vi "Coloring Doppler Demo.vi"() -> ()   [LabVIEW 2018]
uses:
  user.lib/SpectralRadar.llb/OCT Device.lvclass
  user.lib/SpectralRadar.llb/Probe.lvclass
  user.lib/SpectralRadar.llb/Processing.lvclass
  user.lib/SpectralRadar.llb/Raw Data.lvclass
  user.lib/SpectralRadar.llb/Scan Pattern.lvclass
  user.lib/SpectralRadar.llb/Coloring.lvclass
  user.lib/SpectralRadar.llb/Colored Data.lvclass
  user.lib/SpectralRadar.llb/Coloring Byteorder.ctl
  user.lib/SpectralRadar.llb/Device Camera Preset Selection.ctl
  user.lib/SpectralRadar.llb/LabVIEW Helper.lvlib
  user.lib/SpectralRadar.llb/Processing Parameter Int Selection.ctl
  user.lib/SpectralRadar.llb/Colored Data Export Format Selection.ctl
  user.lib/SpectralRadar.llb/set Complex Scan Output.vi
  user.lib/SpectralRadar.llb/Colorscheme Selection.ctl
  user.lib/SpectralRadar.llb/Complex Data.lvclass
  user.lib/SpectralRadar.llb/Doppler Processing.lvclass
  user.lib/SpectralRadar.llb/set Doppler Phase Output.vi
  user.lib/SpectralRadar.llb/set Doppler Amplitude Output.vi
  user.lib/SpectralRadar.llb/Doppler Property Int.ctl
  user.lib/SpectralRadar.llb/Data.lvclass
panel:
  in  "Averaging Z":i32=1
  in  "Averaging X":i32=2 min=2 max=20 step=1
  in  "Min Signal [dB]":sgl(slide)=1.4419259 min=-20 max=120 scale=-20.0..120.0
  in  "Doppler Boundaries":cluster{sgl, sgl}(slide)={1.4419259, -0.7006223} scale=-3.1415..3.1415
  in  "Save Button":bool
  in  "File Name":path
  in  "Display On/Off":bool=TRUE
  in  "Range":dbl=1.0
  in  "Color Table Selection":T1
  out "Averaged Frame Rate":dbl=6.134969234466553 format="%#_3g"
  out "Current Frame Rate":dbl=6.134969234466553 format="%#_3g"
  in  "Boundries":cluster{sgl, sgl}(slide)={76.65738, 42.00557} scale=-20.0..120.0
  out "Image":T2(plugin-control)
  in  "stop":bool
  in  "AScans":i32=1024
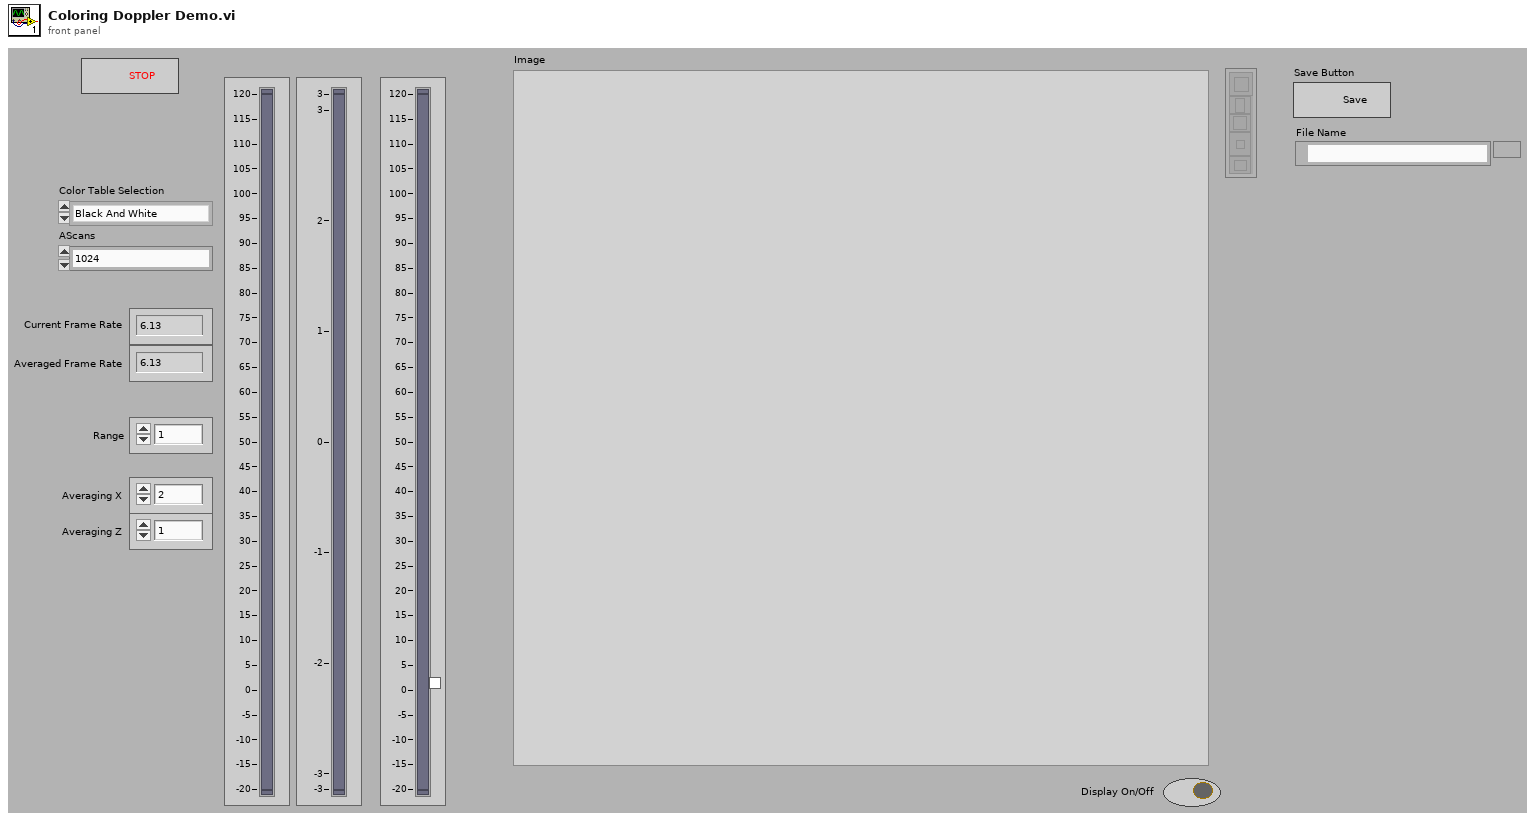
[diagram p1: front panel]
types:
  T1 = typedef "Coloring.lvclass/Colorscheme Selection.ctl" = enum16{"Black And White", "Inverted Black And White", "Color", "Black and Orange", "Black and Red", "Doppler Phase Coloring"}
  T2 = typedef "IMAQ Image.ctl" = refnum<image>
  T3 = typedef "Coloring.lvclass/Coloring Byteorder.ctl" = enum16{"RGBA32", "BGRA32", "ARGB32", ""}
  T4 = typedef "Processing.lvclass/Processing Parameter Int Selection.ctl" = enum32{"Spectrum Averaging", "A-Scan Averaging", "B-Scan Averaging", "Zero Padding", "Number of Threads", "Fourier Averaging"}
  T5 = typedef "OCT Device.lvclass/Device Camera Preset Selection.ctl" = enum16{"Default", "Preset 1", "Preset 2", "Preset 3"}
  T6 = typedef "Image Type" = u32
  T7 = enum16{"Asynchronous Continuous", "Asynchronous Finite", "Synchronous"}
  T8 = typedef "Doppler Processing.lvclass/Doppler Property Int.ctl" = enum16{"Doppler Averaging 1", "Doppler Averaging 2"}
  T9 = typedef "Colored Data.lvclass/Colored Data Export Format Selection.ctl" = enum16{"SRM (Spectral Radar Metafile)", "RAW", "BMP", "PNG", "JPG", "PDF", "TIFF"}
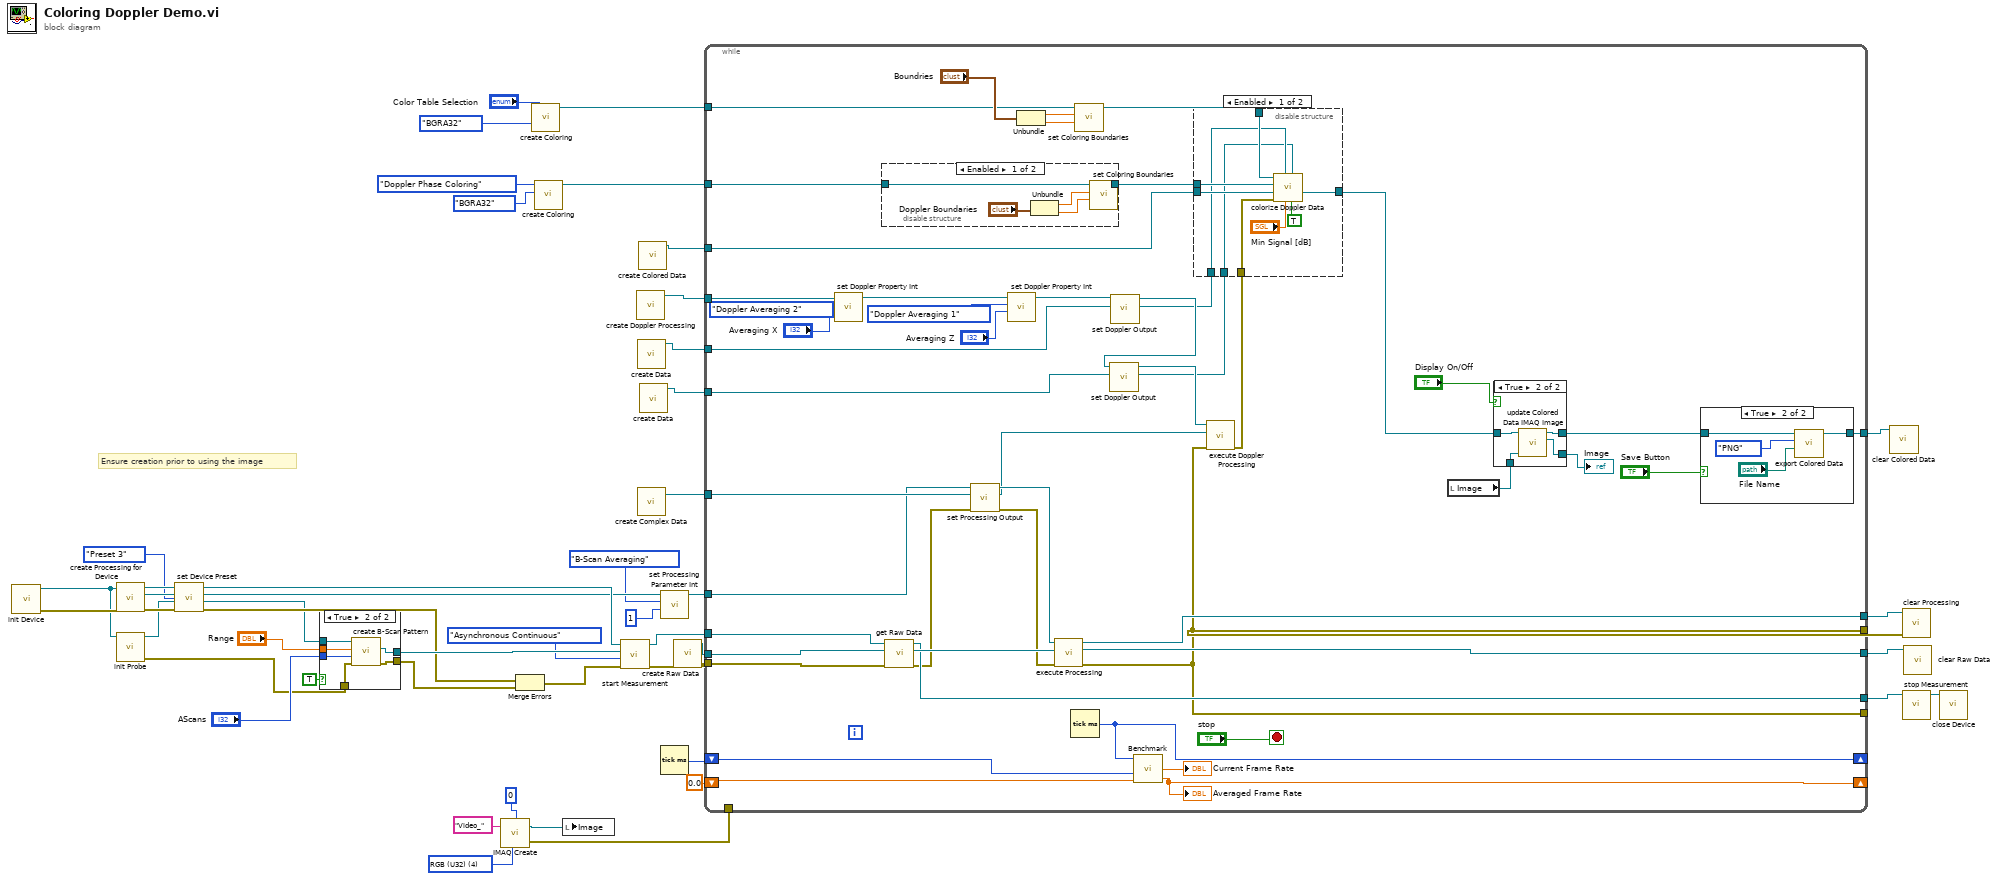
[diagram p0: block diagram]
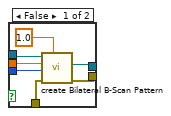
[diagram p2: hidden frame]
diagram:
  w30 = T6 4 items=["Grayscale (U8)", "Grayscale (I16)", "Grayscale (SGL)", "Complex (CSG)", "RGB (U32)", "HSL (U32)", "RGB (U64)", "Grayscale (U16)"] ("Image Type")
  # "Ensure creation prior to using the image"
  n1 = call "init Device.vi"() -> ("error out"=w49:errorcluster, "OCTDevice"=w19:refnum<class "OCT Device.lvclass">)  [unwired: 6 in]
  n2 = call "create Processing for Device.vi"("error in (no error)"=w49, "OCTDevice"=w19) -> ("error out"=w43:errorcluster, "Processing"=w23:refnum<class "Processing.lvclass">, "OCTDevice"=w24:refnum<class "OCT Device.lvclass">)  [unwired: 3 in]
  n3 = call "init Probe.vi"("OCT Device [In]"=w19) -> ("error out"=w32:errorcluster, "OCT Device [Out]"=w20:refnum<class "OCT Device.lvclass">)  [unwired: 4 in, 1 out]
  n4 = call "set Device Preset.vi"("Numeric"=Device_Camera_Preset_Selection."Preset 3" ("Device Camera Preset Selection"), "Probe"=w20, "Processing"=w23, "OCTDevice"=w24) -> ("Probe 2"=w18:refnum<class "Probe.lvclass">, "Processing"=w14:refnum<class "Processing.lvclass">, "OCTDevice out"=w22:refnum<class "OCT Device.lvclass">)  [unwired: 2 in, 1 out]
  n5 = case shown="True" TRUE {
    tunnel: "AScans" -> [w55 w62]
    tunnel: [w54 w61] -> w47
    tunnel: [w53 w60] -> w45
    tunnel: w32 -> [w52 w59]
    tunnel: w18 -> [w56 w58]
    tunnel: "Range" -> [w51 w57]
    frame False {
      n6 = call "create Bilateral B-Scan Pattern.vi"("Rel. Shift Correction"=1.0 ("shift"), "error in (no error)"=w52, "AScans"=w55, "Range"=w51, "Probe"=w56) -> ("error out"=w53:errorcluster, "Scan Pattern"=w54:refnum<class "Scan Pattern.lvclass">)  [unwired: 2 in, 1 out]
    }
    frame True {
      n7 = call "create B-Scan Pattern.vi"("error in (no error)"=w59, "AScans"=w62, "Range"=w57, "Probe"=w58) -> ("error out"=w60:errorcluster, "Scan Pattern"=w61:refnum<class "Scan Pattern.lvclass">)  [unwired: 2 in, 1 out]
    }
  }
  n8 = call "IMAQ Create"("Border Size"=0, "Image Name"="Video_", "Image Type"=w30) -> ("New Image"=w28:T2, "error out"=w4:errorcluster)  [unwired: 2 in]
  n9 = Merge Errors(w43, w45) -> (w44:errorcluster)
  n10 = call "create Coloring.vi"("Color Byte Order"=Coloring_Byteorder."BGRA32", "Color Table Selection"="Color Table Selection") -> ("Coloring"=w27:refnum<class "Coloring.lvclass">)  [unwired: 4 in, 1 out]
  n11 = call "create Coloring.vi"("Color Byte Order"=Coloring_Byteorder."BGRA32", "Color Table Selection"=Colorscheme_Selection."Doppler Phase Coloring") -> ("Coloring"=w8:refnum<class "Coloring.lvclass">)  [unwired: 4 in, 1 out]
  n12 = local write "Image"(w28) -> ()
  n13 = call "start Measurement.vi"("error in (no error)"=w44, "Acquisition Type"=T7."Asynchronous Continuous", "Scan Pattern"=w47, "OCTDevice"=w22) -> ("error out"=w41:errorcluster, "OCTDevice"=w34:refnum<class "OCT Device.lvclass">)  [unwired: 1 in, 1 out]
  n14 = call "create Doppler Processing.vi"() -> ("Doppler Processing"=w6:refnum<class "Doppler Processing.lvclass">)  [unwired: 6 in, 1 out]
  n15 = call "create Data.vi"() -> ("Data"=w2:refnum<class "Data.lvclass">)  [unwired: 6 in, 1 out]
  n16 = call "create Complex Data.vi"() -> ("Complex Data"=w7:refnum<class "Complex Data.lvclass">)  [unwired: 2 in, 1 out]
  n17 = call "create Colored Data.vi"() -> ("Colored Data"=w3:refnum<class "Colored Data.lvclass">)  [unwired: 6 in, 1 out]
  n18 = call "create Data.vi"() -> ("Data"=w1:refnum<class "Data.lvclass">)  [unwired: 6 in, 1 out]
  n19 = call "set Processing Parameter Int.vi"("Value"=1, "Processing Paramter Int Selection"=Processing_Parameter_Int_Selection."B-Scan Averaging", "Processing in"=w14) -> ("Processing out"=w13:refnum<class "Processing.lvclass">)  [unwired: 3 in, 1 out]
  n20 = Tick Count (ms)() -> (millisecond timer value=w26:u32)
  n21 = call "create Raw Data.vi"("error in (no error)"=w41) -> ("error out"=w40:errorcluster, "Raw Data"=w42:refnum<class "Raw Data.lvclass">)  [unwired: 5 in]
  n22 = while {
    tunnel: w42 -> [w110]
    tunnel: w34 -> [w111]
    tunnel: w40 -> [w109]
    tunnel: w13 -> [w86]
    tunnel: [w106] -> w39
    tunnel: [w105] -> w38
    tunnel: [w104] -> w36
    tunnel: [w80] -> w37
    tunnel: [w80] -> _
    tunnel: w27 -> [w79]
    shift-right: [w96] -> _
    shift-left: w26 -> [w98]
    shift-right: [w95] -> _
    shift-left: sgl 0.0 ("AverageFrameRate") -> [w94]
    tunnel: [w90] -> w10
    tunnel: w8 -> [w88]
    tunnel: w7 -> [w87]
    tunnel: w6 -> [w67]
    tunnel: w2 -> [w85]
    tunnel: w1 -> [w83]
    tunnel: w4 -> [_]
    tunnel: w3 -> [w70]
    stop <- "stop" stop-if-true
    n23 = call "set Doppler Property Int.vi"("Value"="Averaging X", "Doppler Property"=Doppler_Property_Int."Doppler Averaging 2", "DopplerProcessing in"=w67) -> ("DopplerProcessing out"=w66:refnum<class "Doppler Processing.lvclass">)  [unwired: 3 in, 1 out]
    n24 = disable-structure shown="Enabled" {
      disable-tunnel: w88 -> [w126 w127]
      disable-tunnel: [w122 w127] -> w75
      frame Enabled {
        n25 = Unbundle("Doppler Boundaries") -> (w124:sgl, w123:sgl)
        n26 = call "set Coloring Boundaries.vi"("Danymic Range High [dB]"=w123, "Dynamic Range Low [dB]"=w124, "Coloring in"=w126) -> ("Coloring out"=w122:refnum<class "Coloring.lvclass">)  [unwired: 3 in, 1 out]
      }
      frame Disabled {
      }
    }
    n27 = call "get Raw Data.vi"("error in (no error)"=w109, "RawData in"=w110, "OCTDevice in"=w111) -> ("error out"=w103:errorcluster, "RawData out"=w107:refnum<class "Raw Data.lvclass">, "OCTDevice out"=w104:refnum<class "OCT Device.lvclass">)  [unwired: 2 in]
    n28 = call-poly "set Processing Output.vi"("error in (no error)"=w103, "Complex Data in"=w87, "Processing"=w86) -> ("error out"=w101:errorcluster, "Complex Data out"=w81:refnum<class "Complex Data.lvclass">, "Processing"=w108:refnum<class "Processing.lvclass">)  [unwired: 2 in]
    n29 = call "set Doppler Property Int.vi"("Value"="Averaging Z", "Doppler Property"=Doppler_Property_Int."Doppler Averaging 1", "DopplerProcessing in"=w66) -> ("DopplerProcessing out"=w69:refnum<class "Doppler Processing.lvclass">)  [unwired: 3 in, 1 out]
    n30 = Unbundle("Boundries") -> (w78:sgl, w77:sgl)
    n31 = call "execute Processing.vi"("error in (no error)"=w101, "Raw Data"=w107, "Processing"=w108) -> ("error out"=w80:errorcluster, "Raw Data"=w106:refnum<class "Raw Data.lvclass">, "Processing"=w105:refnum<class "Processing.lvclass">)  [unwired: 2 in]
    n32 = Tick Count (ms)() -> (millisecond timer value=w96:u32)
    n33 = call "set Coloring Boundaries.vi"("Danymic Range High [dB]"=w77, "Dynamic Range Low [dB]"=w78, "Coloring in"=w79) -> ("Coloring out"=w76:refnum<class "Coloring.lvclass">)  [unwired: 3 in, 1 out]
    n34 = call-poly "set Doppler Output.vi"("Data in"=w85, "DopplerProcessing in"=w69) -> ("Data out"=w74:refnum<class "Data.lvclass">, "DopplerProcessing out"=w84:refnum<class "Doppler Processing.lvclass">)  [unwired: 3 in, 1 out]
    n35 = call-poly "set Doppler Output.vi"("Data in"=w83, "DopplerProcessing in"=w84) -> ("Data out"=w73:refnum<class "Data.lvclass">, "DopplerProcessing out"=w82:refnum<class "Doppler Processing.lvclass">)  [unwired: 3 in, 1 out]
    n36 = call "Benchmark.vi"("Last Frame Rate"=w94, "TimeStart"=w98, "TimeFinish"=w96) -> ("AverageFrameRate"=w95:sgl, "FrameRate"=→"Current Frame Rate":sgl)  [unwired: 1 in, 1 out]
    "Averaged Frame Rate" <- w95
    n37 = call "execute Doppler Processing.vi"("error in (no error)"=w80, "Complex Data in"=w81, "DopplerProcessing in"=w82) -> ("error out"=w72:errorcluster)  [unwired: 2 in, 2 out]
    n38 = disable-structure shown="Enabled" {
      disable-tunnel: w76 -> [w120 _]
      disable-tunnel: w75 -> [w119 _]
      disable-tunnel: w70 -> [w118 w121]
      disable-tunnel: w74 -> [w117 _]
      disable-tunnel: w73 -> [w116 _]
      disable-tunnel: w72 -> [w115 _]
      disable-tunnel: [w114 w121] -> w71
      frame Enabled {
        n39 = call "colorize Doppler Data.vi"("Transpose"=TRUE, "Phase Data"=w116, "Min Signal [dB]"="Min Signal [dB]", "Amplitude Data"=w117, "error in (no error)"=w115, "Colored Data"=w118, "Phase Coloring in"=w119, "Amplitude Coloring in"=w120) -> ("Colored Data out"=w114:refnum<class "Colored Data.lvclass">)  [unwired: 3 out]
      }
      frame Disabled {
      }
    }
    n40 = local read "Image"() -> (w100:T2)
    n41 = case shown="True" "Display On/Off" {
      tunnel: w100 -> [w134 w138]
      tunnel: [w133 w137] -> w91
      tunnel: [w134 w136] -> w92
      tunnel: w71 -> [w133 w135]
      frame False {
      }
      frame True {
        n42 = call "update Colored Data IMAQ Image.vi"("Image in"=w138, "Colored Data"=w135) -> ("Image out"=w136:T2, "Colored Data"=w137:refnum<class "Colored Data.lvclass">)  [unwired: 3 in, 1 out]
      }
    }
    "Image" <- w92
    n43 = case shown="True" "Save Button" {
      tunnel: w91 -> [w128 w129]
      tunnel: [w128 w132] -> w90
      frame False {
      }
      frame True {
        n44 = call "export Colored Data.vi"("File Name"="File Name", "Colored Data Export Format Selection"=Colored_Data_Export_Format_Selection."PNG", "Colored Data in"=w129) -> ("Colored Data out"=w132:refnum<class "Colored Data.lvclass">)  [unwired: 3 in, 1 out]
      }
    }
  }
  n45 = call "clear Colored Data.vi"("Colored Data"=w10) -> ()  [unwired: 6 in, 1 out]
  n46 = call "clear Processing.vi"("error in (no error)"=w37, "Processing"=w38) -> ()  [unwired: 5 in, 1 out]
  n47 = call "stop Measurement.vi"("OCTDevice"=w36) -> ("OCTDevice"=w35:refnum<class "OCT Device.lvclass">)  [unwired: 5 in, 1 out]
  n48 = call "clear Raw Data.vi"("Raw Data"=w39) -> ()  [unwired: 6 in, 1 out]
  n49 = call "close Device.vi"("OCTDevice"=w35) -> ()  [unwired: 6 in, 1 out]
